vi "SDF Small Gasifierl HMI - Manual Control Page.vi"() -> ()   [LabVIEW 2013]
uses:
  <vilib>/NI/Current Value Table/DataTypes/Double_Read.vi
  <vilib>/NI/Current Value Table/Type to Enum.vi
  <vilib>/NI/Current Value Table/DataTypes/Double_Type To Enum.vi
  <vilib>/NI/Current Value Table/FGVs/CVT Globals.vi
  <vilib>/NI/Current Value Table/FGVs/Tag Memory.vi
  <vilib>/NI/Current Value Table/Memory Block.vi
  <vilib>/NI/Current Value Table/DataTypes/Double_Memory Block.vi
  <vilib>/NI/Current Value Table/Current Value Table.lvlib
panel:
  out "TI-101":dbl
  in  "To Back":bool caption="Caption"
  in  "To CVT Viewer":bool caption="Caption"
  in  "To Alarm Display":bool caption="Caption"
  in  "Stop":bool caption="Caption"
  in  "To Machine Control":bool caption="Caption"
  in  "Enable Manual Control":bool
  out "Page's Title":string="Manual Control"
  # "Home"
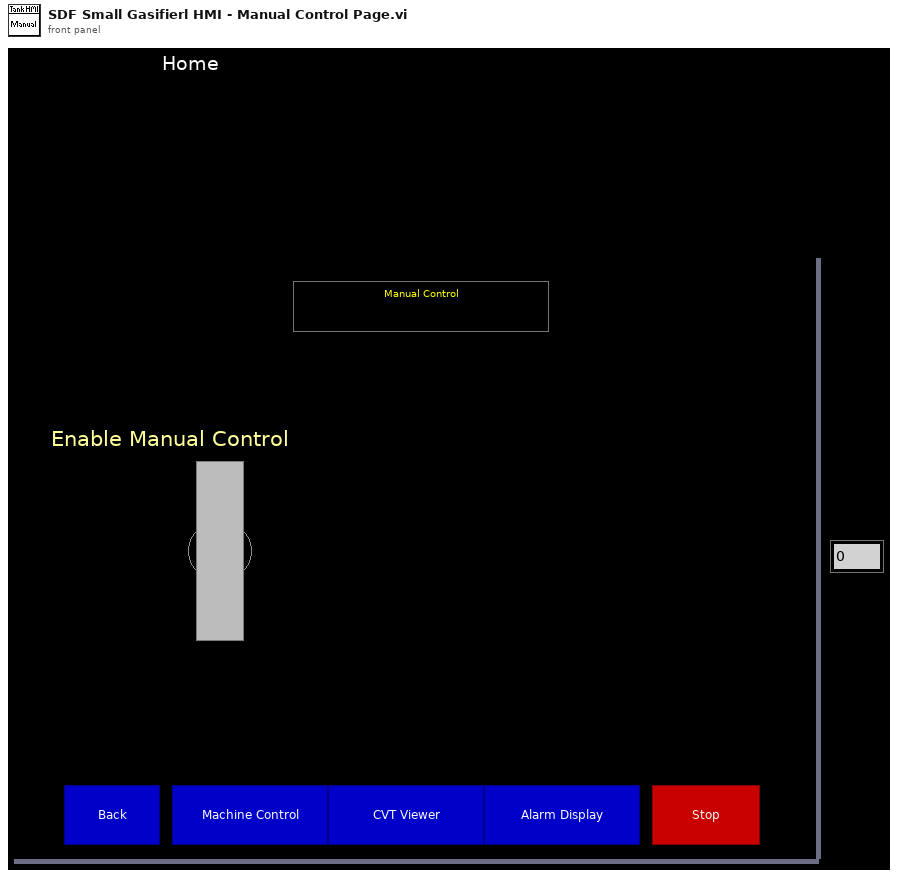
[diagram p1: front panel]
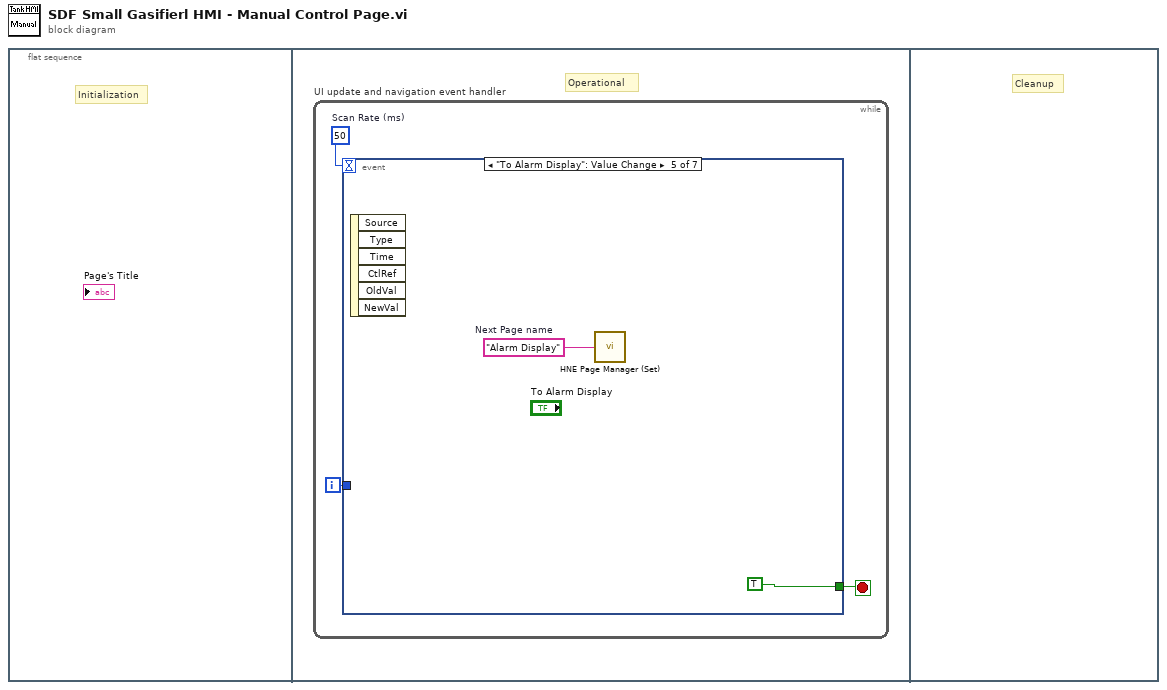
[diagram p0: block diagram]
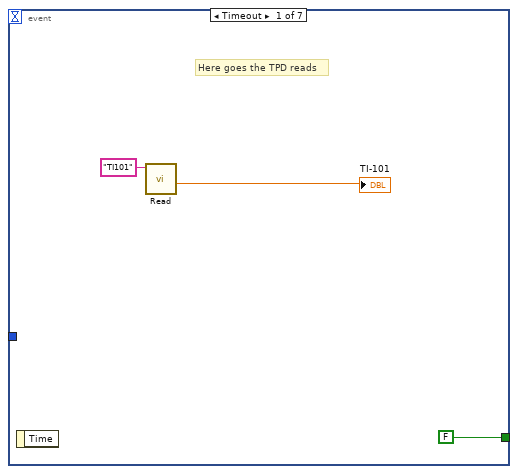
[diagram p2: hidden frame]
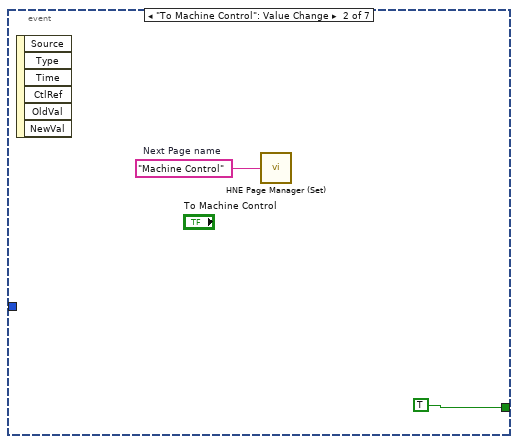
[diagram p3: hidden frame]
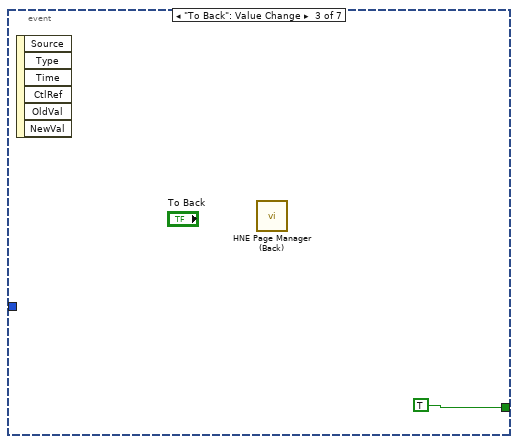
[diagram p4: hidden frame]
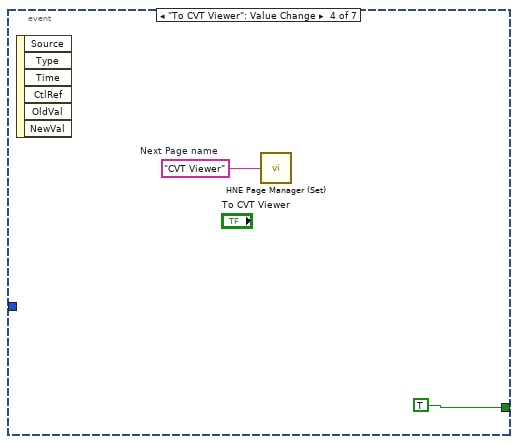
[diagram p5: hidden frame]
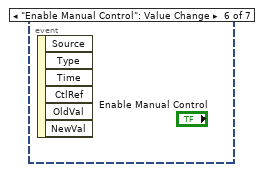
[diagram p6: hidden frame]
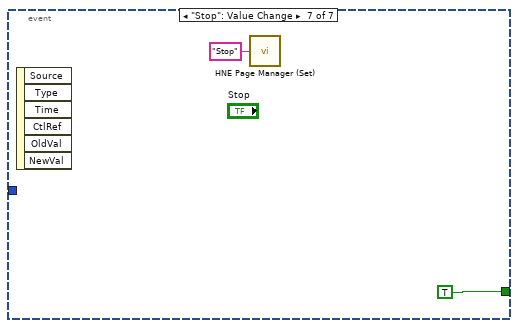
[diagram p7: hidden frame]
diagram:
  n1 = flat-sequence {
    frame #0 {
      # "Initialization"
    }
    frame #1 {
      # "Operational"
      n2 = while "UI update and navigation event handler" {
        i -> [w2]
        stop <- w3 stop-if-true
        w1 = 50  # Scan Rate (ms)
        n3 = event shown="[4] \"To Alarm Display\": Value Change" {
          selector: _ -> [_ _ _ _ _ _ _]
          dyn-events: _ -> [_ _ _ _ _ _ _]
          timeout: w1 -> [_ _ _ _ _ _ _]
          tunnel: [FALSE ("Page Name") TRUE ("Page Name") TRUE ("Page Name") TRUE ("Page Name") TRUE ("Page Name") _ TRUE ("Page Name")] -> w3
          tunnel: w2 -> [_ _ _ _ _ _ _]
          event Timeout {
            # "Here goes the TPD reads"
            n4 = event-data() -> ()  [unwired: 1 in, 1 out]
            n5 = call-poly <vilib>:"Read.vi"("Tag Name"="TI101") -> ("Value"=→"TI-101":dbl)  [unwired: 9 in, 1 out]
          }
          event "To Machine Control": Value Change {
            w8 = "Machine Control"  # Next Page name
            n6 = event-data() -> ()  [unwired: 1 in, 6 out]
            n7 = call <userlib>:"HNE Page Manager (Set).vi"("Next Page"=w8) -> ()  [unwired: 4 in, 1 out]
          }
          event "To Back": Value Change {
            n8 = event-data() -> ()  [unwired: 1 in, 6 out]
            n9 = call <userlib>:"HNE Page Manager (Back).vi"() -> ()  [unwired: 5 in, 1 out]
          }
          event "To CVT Viewer": Value Change {
            w11 = "CVT Viewer"  # Next Page name
            n10 = event-data() -> ()  [unwired: 1 in, 6 out]
            n11 = call <userlib>:"HNE Page Manager (Set).vi"("Next Page"=w11) -> ()  [unwired: 4 in, 1 out]
          }
          event "To Alarm Display": Value Change {
            w13 = "Alarm Display"  # Next Page name
            n12 = event-data() -> ()  [unwired: 1 in, 6 out]
            n13 = call <userlib>:"HNE Page Manager (Set).vi"("Next Page"=w13) -> ()  [unwired: 4 in, 1 out]
          }
          event "Enable Manual Control": Value Change {
            n14 = event-data() -> ()  [unwired: 1 in, 6 out]
          }
          event "Stop": Value Change {
            n15 = event-data() -> ()  [unwired: 1 in, 6 out]
            n16 = call <userlib>:"HNE Page Manager (Set).vi"("Next Page"="Stop") -> ()  [unwired: 4 in, 1 out]
          }
        }
      }
    }
    frame #2 {
      # "Cleanup"
    }
  }
